vi "Read Configuration File.vi"(8 "error in (no error)":errorcluster, 11 "Inst.Krohn-Hite-7008 in":refnum<class "Inst.Krohn-Hite-7008.lvclass">) -> (0 "error out":errorcluster, 3 "Inst.Krohn-Hite-7008 out":refnum<class "Inst.Krohn-Hite-7008.lvclass">)   [LabVIEW 2019, in "Inst.KH7008.lvlib" / "Inst.Krohn-Hite-7008.lvclass"]
uses:
  Inst.Krohn-Hite-7008.lvclass
  <userlib>/LevyLab/Instrument Framework/Instrument Types/Amplifier/Instrument.Amplifier.lvclass
  <userlib>/LevyLab/Configuration/Configuration.lvclass
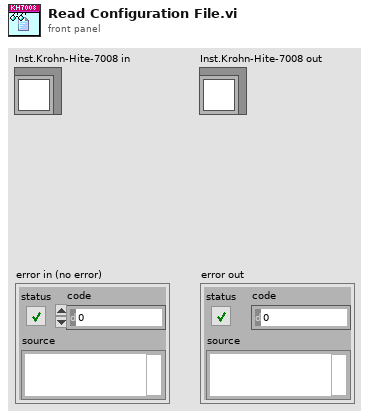
[diagram p1: front panel]
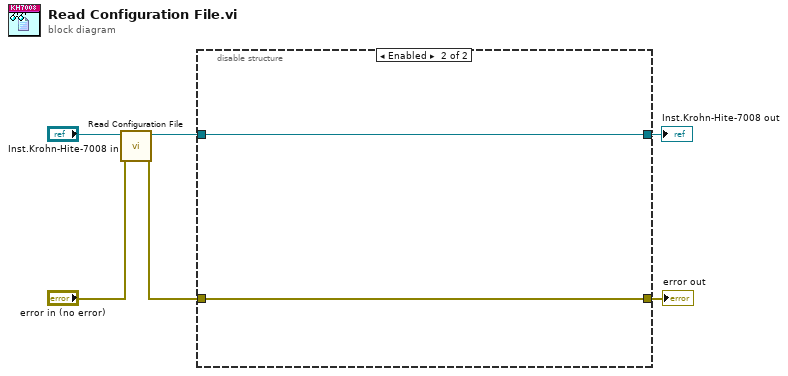
[diagram p0: block diagram]
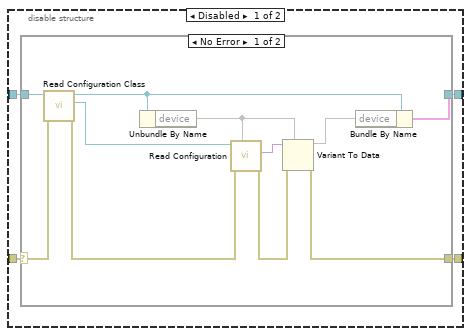
[diagram p2: hidden frame]
diagram:
  n1 = call-parent "Read Configuration File.vi"("error in (no error)"="error in (no error)", "Instrument in"="Inst.Krohn-Hite-7008 in") -> ("error out"=w1:errorcluster, "Instrument out"=w3:refnum<class "Inst.Krohn-Hite-7008.lvclass">)  [unwired: 8 in]
  n2 = disable-structure shown="Enabled" {
    disable-tunnel: [w10 w25] -> w6
    disable-tunnel: [w9 w24] -> w5
    disable-tunnel: w3 -> [w8 w25]
    disable-tunnel: w1 -> [w7 w24]
    frame Disabled {
      n3 = case shown="No Error" w7 {
        selector: w7 -> [w18 w23]
        tunnel: w8 -> [w20 w22]
        tunnel: [w14 w22] -> w10
        tunnel: [w19 w23] -> w9
        frame No Error {
          n4 = call <userlib>:"Read Configuration Class.vi"("error in (no error)"=w18, "Instrument in"=w20) -> ("error out"=w15:errorcluster, "Configuration"=w13:refnum<class "Configuration.lvclass">, "Instrument out"=w12:refnum<class "Inst.Krohn-Hite-7008.lvclass">)  [unwired: 7 in]
          n5 = Unbundle By Name(w12) -> ("device"=w17)
          n6 = call <userlib>:"Read Configuration.vi"("INI Fomatted Cluster Type"=w17, "error in (no error)"=w15, "Configuration in"=w13) -> ("error out"=w21:errorcluster, "Configuration"=w16:variant)  [unwired: 6 in, 1 out]
          n7 = Variant To Data(error in=w21, type=w17, Variant=w16) -> (data=w11, error out=w19:errorcluster)
          n8 = Bundle By Name(cluster=w12, "device"=w11) -> (w14:cluster{})
        }
        frame Error {
        }
      }
    }
    frame Enabled {
    }
  }
  "Inst.Krohn-Hite-7008 out" <- w6
  "error out" <- w5
